vi "DAQ Init.vi"(0 "Model":string) -> (1 "task out":refnum<k21>, 2 "error out":errorcluster)   [LabVIEW 2023]
uses:
  <vilib>/DAQmx/create/channels.llb/DAQmx Create Channel (DO-Digital Output).vi
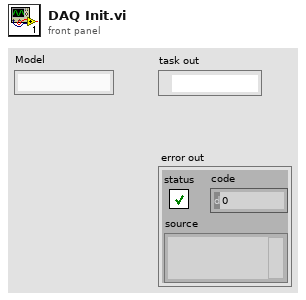
[diagram p1: front panel]
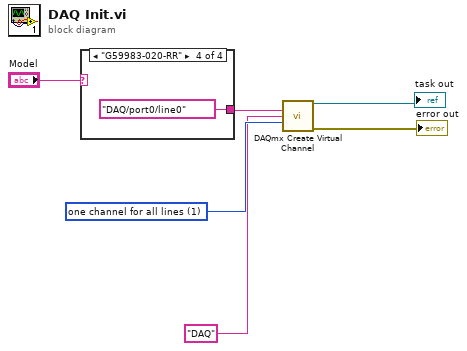
[diagram p0: block diagram]
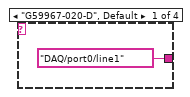
[diagram p2: hidden frame]
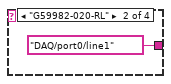
[diagram p3: hidden frame]
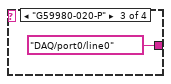
[diagram p4: hidden frame]
diagram:
  w2 = 1 items=["one channel for each line", "one channel for all lines"] ("line grouping")
  n1 = case shown="\"G59983-020-RR\"" "Model" {
    tunnel: [tag "DAQ/port0/line1" ("lines") tag "DAQ/port0/line1" ("lines") tag "DAQ/port0/line0" ("lines") tag "DAQ/port0/line0" ("lines")] -> w5
    frame "G59967-020-D", Default {
    }
    frame "G59982-020-RL" {
    }
    frame "G59980-020-P" {
    }
    frame "G59983-020-RR" {
    }
  }
  n2 = call-poly <vilib>:"DAQmx Create Virtual Channel.vi"("lines"=w5, "name to assign"="DAQ", "line grouping"=w2) -> ("task out"=→"task out":refnum<k21>, "error out"=→"error out":errorcluster)  [unwired: 11 in]
